vi "BrakeStuffs.vi"   [LabVIEW 2014]
uses:
  Support Files/Brake.ctl
  Support Files/Global Data!!!.vi
types:
  T1 = typedef "Brake.ctl" = enum16{"Reset", "Pause", "Engage/Disengage", "Rest"}
  T2 = typedef "WPI_MotorControlDeviceRef.ctl" = cluster{"DeviceStatus":errorcluster, "Type":T3, "PWM":cluster{"Controller":T4, "PWM Channel":T5, "DeadBand":T6}, "CAN":cluster{"Device Number":u8, "Control Mode":T7, "Semaphore":T8, "Max Vout":dbl, "TalonSRX Control Mode":T9}, "Invert":bool, "TransformRef":T10, "InvTransformRef":T10}
  T3 = typedef "WPI_MotorControlType.ctl" = enum16{"PWM", "CAN", "CANTalonSRX"}
  T4 = typedef "FPGA_TypedefDigitalModule.ctl" = enum16{"Controller 1"}
  T5 = typedef "FPGA_DIOPWMChannel.ctl" = enum8{"PWM 0", "PWM 1", "PWM 2", "PWM 3", "PWM 4", "PWM 5", "PWM 6", "PWM 7", "PWM 8", "PWM 9", "PWM MXP 0", "PWM MXP 1", "PWM MXP 2", "PWM MXP 3", "PWM MXP 4", "PWM MXP 5", "PWM MXP 6", "PWM MXP 7", "PWM MXP 8", "PWM MXP 9", "Invalid"}
  T6 = typedef "WPI_PWMDeadband.ctl" = cluster{"Name":string, "maxPositivePwm":i32, "minPositivePwm":i32, "centerPwm":i32, "maxNegativePwm":i32, "minNegativePwm":i32, "angularRange":u16}
  T7 = typedef "WPI_CANJaguar_ControlMode.ctl" = enum8{"Percent VBus", "Current", "Speed", "Position", "Voltage"}
  T8 = typedef "Semaphore RefNum" = refnum<k1>
  T9 = typedef "WPI_CANTalonSRX_APIControlMode.ctl" = enum8{"Percent VBus", "Speed", "Position", "Slave", "Unchanged / Invalid"}
  T10 = typedef "WPI_PWMTransform_ConPane.ctl" = refnum<vi>
  T11 = typedef "WPI_SwitchDevRef.ctl" = cluster{"DevStatus":errorcluster, "DIO Channel":T12, "Controller":T4, "CntIndex":T13, "Normally Closed":bool}
  T12 = typedef "FPGA_DIOChannel.ctl" = enum8{"DIO 0", "DIO 1", "DIO 2", "DIO 3", "DIO 4", "DIO 5", "DIO 6", "DIO 7", "DIO 8", "DIO 9", "DIO MXP 0", "DIO MXP 1", "DIO MXP 2", "DIO MXP 3", "DIO MXP 4", "DIO MXP 5", "DIO MXP 6", "DIO MXP 7", "DIO MXP 8", "DIO MXP 9", "DIO MXP 10", "DIO MXP 11", "DIO MXP 12", "DIO MXP 13", "DIO MXP 14", "DIO MXP 15", "Invalid"}
  T13 = typedef "FPGA_CounterCtrSystemIndex.ctl" = enum8{"Ctr 0", "Ctr 1", "Ctr 2", "Ctr 3", "Ctr 4", "Ctr 5", "Ctr 6", "Ctr 7", "Invalid"}
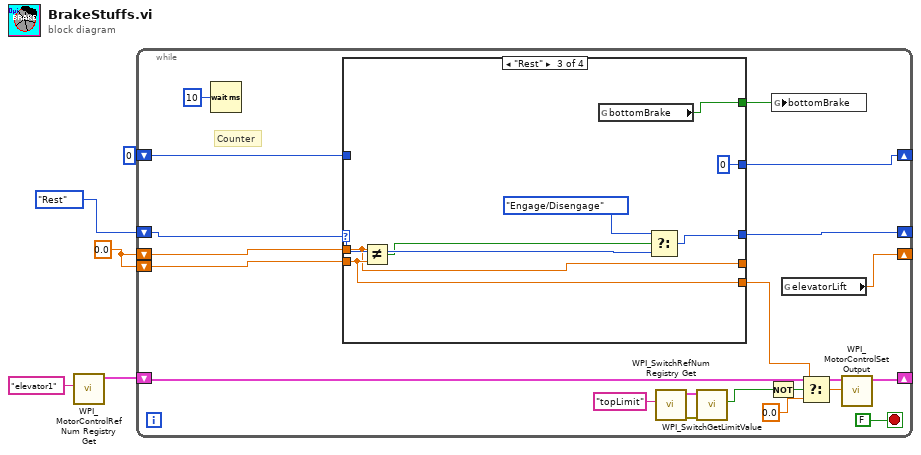
[diagram p0: block diagram]
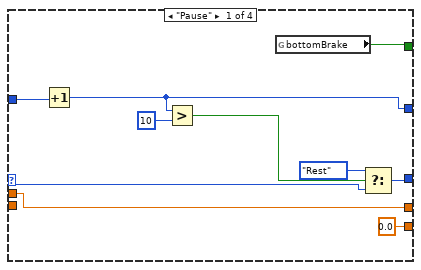
[diagram p2: hidden frame]
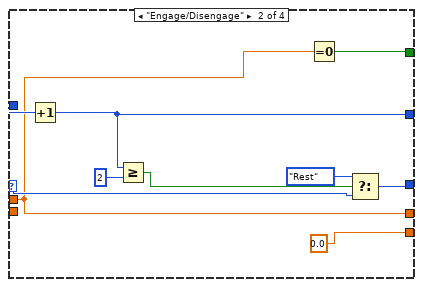
[diagram p3: hidden frame]
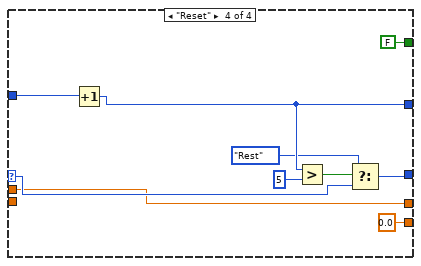
[diagram p4: hidden frame]
diagram:
  w5 = 0.0 ("elevatorLift")
  n1 = call <vilib>:"WPI_MotorControlRefNum Registry Get.vi"("refnum name"="elevator1") -> ("MotorControlDevRef"=w3:T2)  [unwired: 9 in, 1 out]
  n2 = while {
    shift-right: [w25] -> _
    shift-left: Brake."Rest" -> [w6]
    shift-right: [w16] -> _
    shift-left: w5 -> [w24]
    shift-left: w5 -> [w23]
    shift-right: [w21] -> _
    shift-left: 0 ("y") -> [w22]
    shift-right: [w20] -> _
    shift-left: w3 -> [w19]
    stop <- FALSE stop-if-true
    # "Counter"
    n3 = Wait (ms)(milliseconds to wait=u32 10) -> ()  [unwired: 1 out]
    n4 = case shown="\"Rest\"" w6 {
      selector: w6 -> [w31 w44 w53 w57]
      tunnel: [w32 w45 w52 w61] -> w25
      tunnel: w24 -> [w27 w37 w47 w55]
      tunnel: w23 -> [_ _ w49 _]
      tunnel: w22 -> [w35 w41 _ w62]
      tunnel: [w34 w40 0 w59] -> w21
      tunnel: [0.0 ("elevatorLift") 0.0 ("f") w49 0.0 ("elevatorLift")] -> w13
      tunnel: [w29 w39 w48 FALSE ("bottomBrake")] -> w18
      tunnel: [w27 w37 w47 w55] -> _
      frame "Pause" {
        n5 = Increment(x=w35) -> (x+1=w34:i32)
        n6 = Greater?(x=w34, y=10) -> (0:w30:bool)
        n7 = global read "Global Data!!!.vi" "bottomBrake"() -> (w29:bool)
        n8 = Select(t=Brake."Rest", s=w30, f=w31) -> (s? t:f=w32:T1)
      }
      frame "Engage/Disengage" {
        n9 = Increment(x=w41) -> (x+1=w40:i32)
        n10 = Greater Or Equal?(x=w40, y=2) -> (x >= y?=w42:bool)
        n11 = Equal To 0?(x=w37) -> (x = 0?=w39:bool)
        n12 = Select(t=Brake."Rest", s=w42, f=w44) -> (s? t:f=w45:T1)
      }
      frame "Rest" {
        n13 = Not Equal?(x=w47, y=w49) -> (x != y?=w51:bool)
        n14 = global read "Global Data!!!.vi" "bottomBrake"() -> (w48:bool)
        n15 = Select(t=Brake."Engage/Disengage", s=w51, f=w53) -> (s? t:f=w52:T1)
      }
      frame "Reset" {
        n16 = Increment(x=w62) -> (x+1=w59:i32)
        n17 = Greater?(x=w59, y=5) -> (0:w60:bool)
        n18 = Select(t=Brake."Rest", s=w60, f=w57) -> (s? t:f=w61:T1)
      }
    }
    n19 = call <vilib>:"WPI_SwitchRefNum Registry Get.vi"("refnum name"="topLimit") -> ("error out"=w11:errorcluster, "SwitchDevRef"=w10:T11)  [unwired: 9 in]
    n20 = call <vilib>:"WPI_SwitchGetLimitValue.vi"("error in (no error)"=w11, "SwitchDevRef"=w10) -> ("Switch Pressed"=w8:bool)  [unwired: 7 in, 2 out]
    n21 = Not(x=w8) -> (.not. x?=w9:bool)
    n22 = global write "Global Data!!!.vi" "bottomBrake"(w18) -> ()
    n23 = global read "Global Data!!!.vi" "elevatorLift"() -> (w16:dbl)
    n24 = Select(t=w13, s=w9, f=0.0) -> (s? t:f=w14:dbl)
    n25 = call <vilib>:"WPI_MotorControlSetOutput.vi"("Output"=w14, "MotorControlDevRef"=w19) -> ("MotorControlDevRef"=w20:T2)  [unwired: 7 in, 2 out]
  }
